vi "Files_names.vi"(2 "actualSamples\narray":i32[](array[numeric]), 3 "Type of\nmeasurement":u16, 4 "Name root":string, 5 "File location":path) -> (0 "Files path array":path[](array[path]), 1 "Files name array":string[](array[string]))   [LabVIEW 2013]
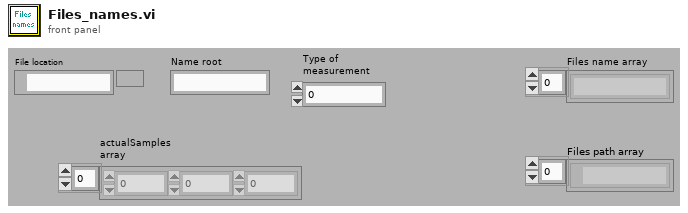
[diagram p1: front panel]
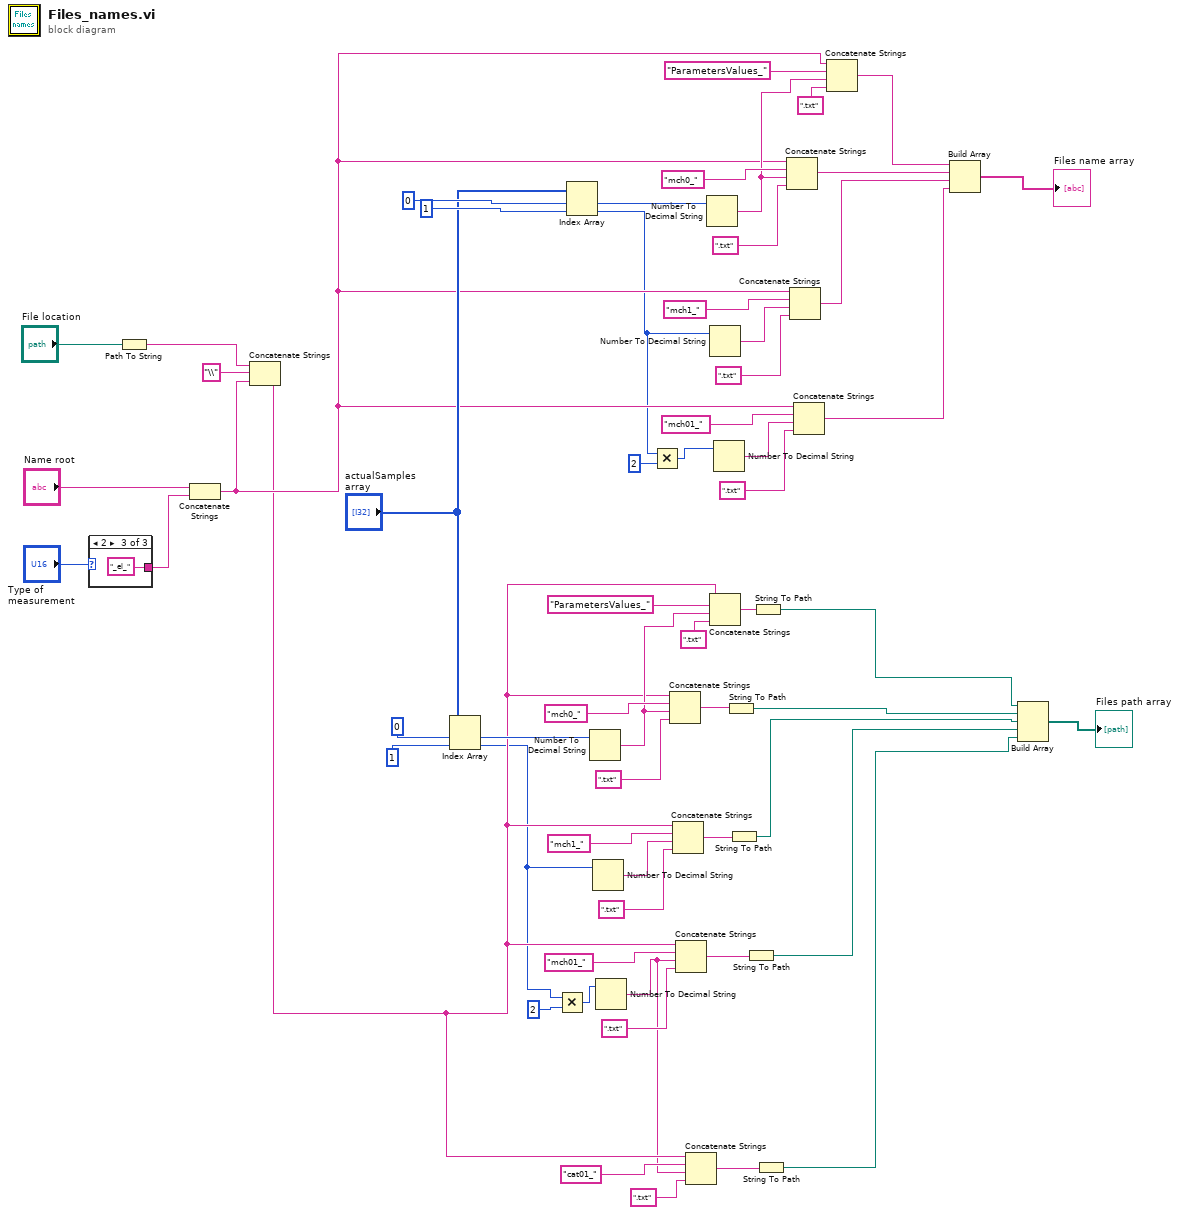
[diagram p0: block diagram]
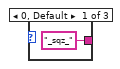
[diagram p2: hidden frame]
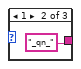
[diagram p3: hidden frame]
diagram:
  n1 = case shown="2" "Type of\nmeasurement" {
    tunnel: ["_sqz_" "_qn_" "_el_"] -> w45
    frame 0, Default {
    }
    frame 1 {
    }
    frame 2 {
    }
  }
  n2 = Path To String(path="File location") -> (string=w30:string)
  n3 = Concatenate Strings("Name root", w45) -> (w13:string)
  n4 = Concatenate Strings(w30, "\\" ("string"), w13) -> (w5:string)
  n5 = Index Array(array="actualSamples\narray", index #1=0 ("index"), index #2=1 ("index")) -> (element #1=w52:i32, element #2=w4:i32)
  n6 = Multiply(x=w4, y=2) -> (x*y=w3:i32)
  n7 = Index Array(array="actualSamples\narray", index #1=0 ("index"), index #2=1 ("index")) -> (element #1=w37:i32, element #2=w12:i32)
  n8 = Number To Decimal String(number=w52) -> (decimal integer string=w44:string)  [unwired: 1 out]
  n9 = Number To Decimal String(number=w4) -> (decimal integer string=w50:string)  [unwired: 1 out]
  n10 = Number To Decimal String(number=w3) -> (decimal integer string=w2:string)  [unwired: 1 out]
  n11 = Multiply(x=w12, y=2) -> (x*y=w11:i32)
  n12 = Concatenate Strings(w5, "mch0_" ("string"), w44, ".txt") -> (w48:string)
  n13 = Concatenate Strings(w5, "mch1_" ("string"), w50, ".txt") -> (w47:string)
  n14 = Concatenate Strings(w5, "mch01_" ("string"), w2, ".txt") -> (w19:string)
  n15 = Concatenate Strings(w5, "cat01_" ("string"), w2, ".txt") -> (w6:string)
  n16 = Number To Decimal String(number=w37) -> (decimal integer string=w33:string)  [unwired: 1 out]
  n17 = Number To Decimal String(number=w12) -> (decimal integer string=w35:string)  [unwired: 1 out]
  n18 = Concatenate Strings(w5, "ParametersValues_" ("string"), w44, ".txt" ("string")) -> (w59:string)
  n19 = Number To Decimal String(number=w11) -> (decimal integer string=w16:string)  [unwired: 1 out]
  n20 = String To Path(string=w48) -> (path=w24:path)
  n21 = String To Path(string=w47) -> (path=w25:path)
  n22 = String To Path(string=w19) -> (path=w18:path)
  n23 = String To Path(string=w59) -> (path=w23:path)
  n24 = String To Path(string=w6) -> (path=w1:path)
  n25 = Concatenate Strings(w13, "mch0_" ("string"), w33, ".txt") -> (w29:string)
  n26 = Concatenate Strings(w13, "mch1_" ("string"), w35, ".txt") -> (w27:string)
  n27 = Concatenate Strings(w13, "mch01_" ("string"), w16, ".txt") -> (w14:string)
  n28 = Concatenate Strings(w13, "ParametersValues_" ("string"), w33, ".txt" ("string")) -> (w28:string)
  n29 = Build Array(w28, w29, w27, w14) -> (→"Files name array":string[])
  n30 = Build Array(w23, w24, w25, w18, w1) -> (→"Files path array":path[])
